vi "CSM - Timestamp to API String Arguments.vi"(7 "Format(Empty to use UTC)":string, 8 "UTC? (F)":bool, 11 "Timestamp (now)":timestamp) -> (3 "CSM Timestamp Argument":string)   [LabVIEW 2017, in "API String Arguments Support.lvlib"]
uses:
  API String Arguments Support.lvlib
  <userlib>/_NEVSTOP/Communicable State Machine(CSM)/Communicable State Machine.lvlib
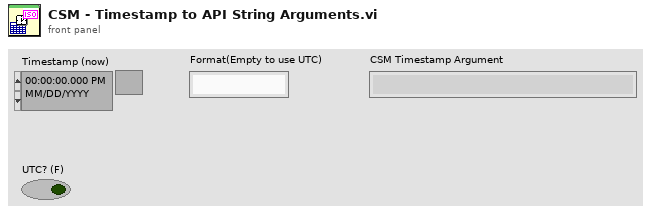
[diagram p1: front panel]
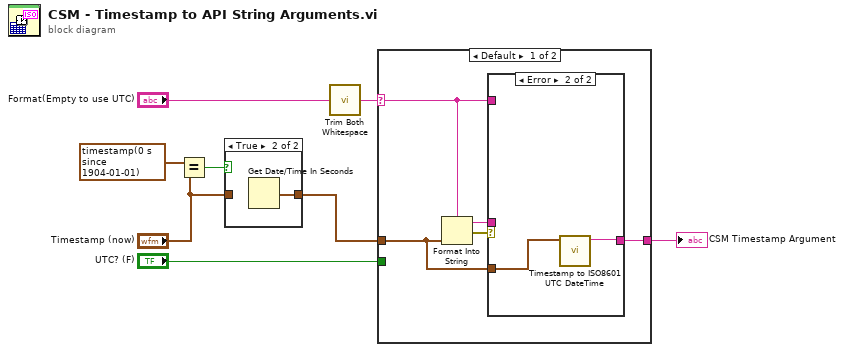
[diagram p0: block diagram]
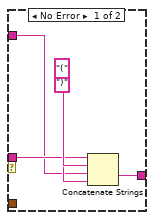
[diagram p3: hidden frame]
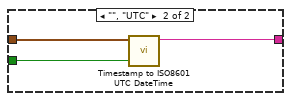
[diagram p4: hidden frame]
diagram:
  n1 = Equal?(x=timestamp(0 s since 1904-01-01), y="Timestamp (now)") -> (x = y?=w3:bool)
  n2 = case shown="True" w3 {
    tunnel: [w9 w10] -> w1
    tunnel: "Timestamp (now)" -> [w9 _]
    frame False {
    }
    frame True {
      n3 = Get Date/Time In Seconds() -> (seconds since 1Jan1904=w10:timestamp)
    }
  }
  n4 = call <userlib>:"Trim Both Whitespace.vi"("string"="Format(Empty to use UTC)") -> ("trimmed string"=w5:string)  [unwired: 1 in]
  n5 = case shown="Default" w5 {
    selector: w5 -> [w14 _]
    tunnel: w1 -> [w11 w25]
    tunnel: "UTC? (F)" -> [_ w24]
    tunnel: [w13 w23] -> w7
    frame Default {
      n6 = Format Into String(format string=w14, w11) -> (resulting string=w15:string, error out=w12:errorcluster)  [unwired: 2 in]
      n7 = case shown="Error" w12 {
        tunnel: w15 -> [w18 _]
        tunnel: w14 -> [w17 _]
        tunnel: [w16 w22] -> w13
        tunnel: w11 -> [_ w21]
        frame No Error {
          n8 = Concatenate Strings(w18, "(" ("string"), w17, ")" ("string")) -> (w16:string)
        }
        frame Error {
          n9 = call <vilib>:"Timestamp to ISO8601 UTC DateTime.vi"("Timestamp (now)"=w21) -> ("ISO8601 UTC DateTime"=w22:string)  [unwired: 10 in]
        }
      }
    }
    frame "", "UTC" {
      n10 = call <vilib>:"Timestamp to ISO8601 UTC DateTime.vi"("UTC? (F)"=w24, "Timestamp (now)"=w25) -> ("ISO8601 UTC DateTime"=w23:string)  [unwired: 9 in]
    }
  }
  "CSM Timestamp Argument" <- w7
